vi "flow_queue_timeout.vi"(6 "timeout?":bool, 7 "local command":string, 8 "error in (no error)":errorcluster caption="エラー入力（エラーなし）", 9 "parameter in":variant, 10 "command in":string) -> (0 "error out":errorcluster caption="エラー出力", 1 "parameter out":variant, 2 "command out":string)   [LabVIEW 2015]
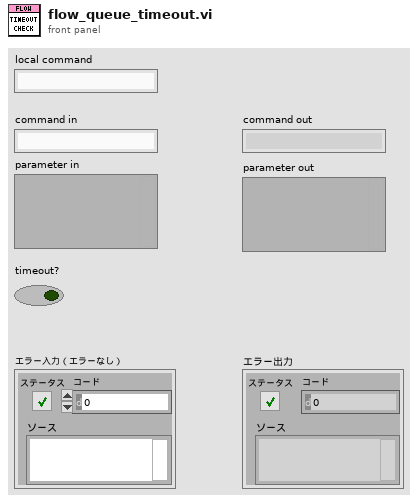
[diagram p1: front panel]
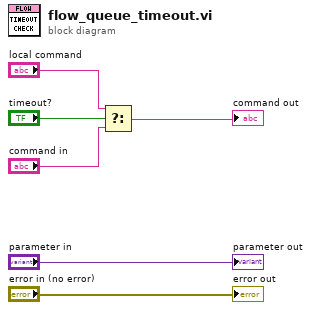
[diagram p0: block diagram]
diagram:
  n1 = Select(t="local command", s="timeout?", f="command in") -> (s? t:f=→"command out":string)
  "error out" <- "error in (no error)"
  "parameter out" <- "parameter in"
